vi "CRYReplace ItemSymbols.vi"(11 "Listbox In":refnum<vi>) -> ()   [LabVIEW 2013]
uses:
  Global/CRYCurve Library Global.vi
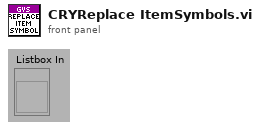
[diagram p1: front panel]
types:
  T1 = typedef "CRYImageData.ctl" = cluster{"image type":i32, "image depth":i32, "image":u8[], "mask":u8[], "colors":u32[], "Rectangle":cluster{"left":i16, "top":i16, "right":i16, "bottom":i16}}
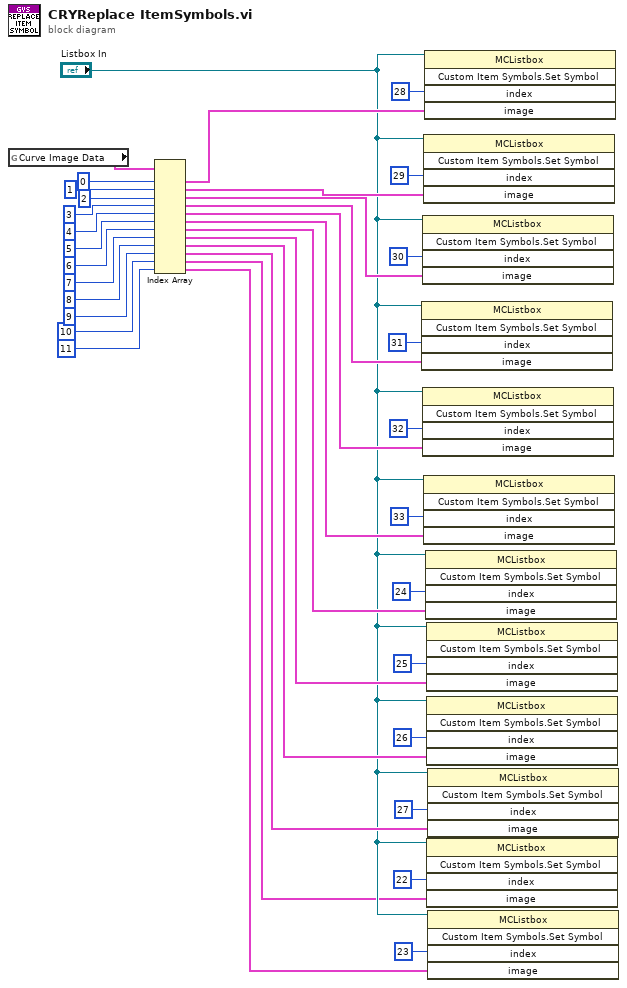
[diagram p0: block diagram]
diagram:
  n1 = global read "CRYCurve Library Global.vi" "Curve Image Data"() -> (w1:T1[])
  n2 = Index Array(array=w1, index #1=0 ("index"), index #2=1 ("index"), index #3=2 ("index"), index #4=3 ("index"), index #5=4 ("index"), index #6=5 ("index"), index #7=6 ("index"), index #8=7 ("index"), index #9=8 ("index"), index #10=9 ("index"), index #11=10 ("index"), index #12=11 ("index")) -> (element #1=w26:T1, element #2=w25:T1, element #3=w24:T1, element #4=w23:T1, element #5=w22:T1, element #6=w21:T1, element #7=w16:T1, element #8=w15:T1, element #9=w10:T1, element #10=w9:T1, element #11=w3:T1, element #12=w2:T1)
  n3 = invoke class="MCListbox" method="Custom Item Symbols.Set Symbol"(reference="Listbox In", "index"=31 ("Index"), "image"=w23) -> ()  [unwired: 2 in, 5 out]
  n4 = invoke class="MCListbox" method="Custom Item Symbols.Set Symbol"(reference="Listbox In", "index"=30 ("Index"), "image"=w24) -> ()  [unwired: 2 in, 5 out]
  n5 = invoke class="MCListbox" method="Custom Item Symbols.Set Symbol"(reference="Listbox In", "index"=32 ("Index"), "image"=w22) -> ()  [unwired: 2 in, 5 out]
  n6 = invoke class="MCListbox" method="Custom Item Symbols.Set Symbol"(reference="Listbox In", "index"=29 ("Index"), "image"=w25) -> ()  [unwired: 2 in, 5 out]
  n7 = invoke class="MCListbox" method="Custom Item Symbols.Set Symbol"(reference="Listbox In", "index"=33 ("Index"), "image"=w21) -> ()  [unwired: 2 in, 5 out]
  n8 = invoke class="MCListbox" method="Custom Item Symbols.Set Symbol"(reference="Listbox In", "index"=28 ("Index"), "image"=w26) -> ()  [unwired: 2 in, 5 out]
  n9 = invoke class="MCListbox" method="Custom Item Symbols.Set Symbol"(reference="Listbox In", "index"=24 ("Index"), "image"=w16) -> ()  [unwired: 2 in, 5 out]
  n10 = invoke class="MCListbox" method="Custom Item Symbols.Set Symbol"(reference="Listbox In", "index"=25 ("Index"), "image"=w15) -> ()  [unwired: 2 in, 5 out]
  n11 = invoke class="MCListbox" method="Custom Item Symbols.Set Symbol"(reference="Listbox In", "index"=26 ("Index"), "image"=w10) -> ()  [unwired: 2 in, 5 out]
  n12 = invoke class="MCListbox" method="Custom Item Symbols.Set Symbol"(reference="Listbox In", "index"=22 ("Index"), "image"=w3) -> ()  [unwired: 2 in, 5 out]
  n13 = invoke class="MCListbox" method="Custom Item Symbols.Set Symbol"(reference="Listbox In", "index"=27 ("Index"), "image"=w9) -> ()  [unwired: 2 in, 5 out]
  n14 = invoke class="MCListbox" method="Custom Item Symbols.Set Symbol"(reference="Listbox In", "index"=23 ("Index"), "image"=w2) -> ()  [unwired: 2 in, 5 out]
